vi "DopplerScale.vi"(6 "FFT Length":i32=512, 7 "Header In":T2={"header info"={"Header"="", "Head length"=0}, "A/D info"={"# rf points per line"=0, "# lines per scan"=0, "sample rate MHz"=0, "# A/D bits"=0, "# bytes per A/D"=0, "TGC Flag"=0, "A/D Type"=""}, "Tranducer Info"={"bandwidth"=0.0, "center freq"=0.0, "start freq"=0.0, "ID"=0}, "Scan Info"={"delay"=0.0, "pivot distance"=0.0, "sector scan angle"=0.0, "operator"="", "Scan Mode"="", "location"=""}, "Time/Date Info"={"date"="", "time"=""}, "RF Info"={"RF file name"="", "RF file att"="", "RF cal file name"="", "RF cal file att"=""}, "Patient Info"={"ID"="", "extended ID"="", "age"=0, "sex"="", "previously\nscanned"="", "PSA"=0.0, "LOS"=1, "Ethnicty 2"=3, "Race"=3}, "Tissue Type"={"organ"=0, "disease type"=0, "disease location"=0, "IQ_pts"=0, "RcvBuffer"=0, "RcvFrame"=0, "IQBuff"=0, "IQFrame"=0, "IQPage"=0}, "Votage scaling"={"Digitizer (dB)"=0.0, "Gain (dB)"=0.0, "Atten (dB)"=0.0}, "Comment"="", "Misc Info"={"avg num"=0, "c speed"=0, "Div By or SF zones"=0, "XMIT CHS"=0, "RCV CHS"=0, "Xmit angle"=0.0}, "Therapy Parameters"={"Theraputic Freq (MHz)"=0.0, "Time on (s)"=0.0, "Therapy amplitude (mV)"=0.0, "Lines Before"=0, "Lines After"=0}, "Scan Settings"={"Energy (uJ or V)"=0, "Damp (Ohm) or Fc"=0, "HP Filt (KHz)"=0, "LP Filt (MHz)"=0, "Gain (db)"=0, "prf (kHz)"=0.0, "Distance between\nscan lines (um)"=0, "Distance between\nscan planes (um)"=0, "Scan line gap (um)"=0.0, "Scan plane gap (um)"=0.0}, "Compression Parameters"={"F1 (MHz)"=0.0, "F2 (MHz)"=0.0, "% taper"=0.0, "duration"=0.0}, "Patient Info Xtra"={"First Name"="", "Last Name"="", "Notes"=""}, "ROI Box"=[0, 0, 0, 0]} {"Compression Parameters"."% taper" min=50 max=1000 format="%.2f"; "Compression Parameters"."F2 (MHz)" format="%.3f"; "Compression Parameters"."F1 (MHz)" format="%.3f"; "Scan Settings"."prf (kHz)" format="%.2f"; "Therapy Parameters"."Therapy amplitude (mV)" min=50 max=1000 format="%.2f"; "Therapy Parameters"."Time on (s)" format="%.3f"; "Therapy Parameters"."Theraputic Freq (MHz)" format="%.3f"; "Patient Info"."Race" items=["Am Ind or Alaska", "Asian", "Hawaiian, Pac Isl", "Black or Afr Amer", "White", "more than one race", "unknown"]; "Patient Info"."Ethnicty 2" items=["Hispanic", "Non-Hispanic", "unknown"]; "Patient Info"."LOS" items=["1", "2", "3", "4", "5"]; "Patient Info"."PSA" format="%.1f"; "Scan Info"."delay" format="%.2f"; "Scan Info"."pivot distance" format="%.2f"; "Scan Info"."sector scan angle" format="%.2f"; "Tranducer Info"."bandwidth" format="%.2f"; "Tranducer Info"."center freq" format="%.2f"; "Tranducer Info"."start freq" format="%.2f"}, 8 "Index(F)/Fd":bool, 9 "PRF1/2":bool=TRUE, 10 "Angle":dbl, 11 "Velocity index in":dbl[][](array[numeric])=array400x128[51200 elements]) -> (0 "output cluster":T1, 1 "slow-time sampling":dbl, 2 "max doppler velocity cm/s":dbl, 3 "Velocity Out":dbl[][](array[numeric]))   [LabVIEW 2022 SP3]
uses:
  Header.ctl
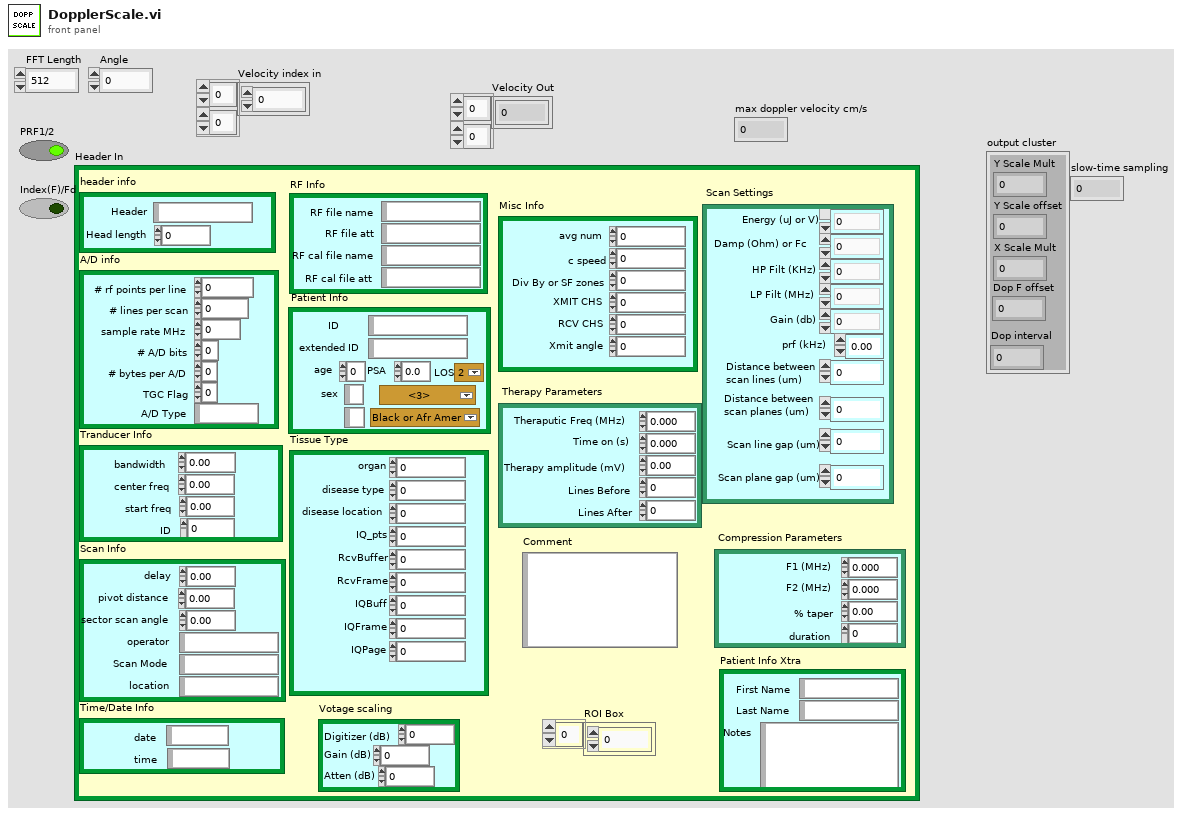
[diagram p1: front panel]
types:
  T1 = cluster{"Y Scale Mult":dbl, "Y Scale offset":dbl, "X Scale Mult":dbl, "Dop F offset":dbl, "Dop interval":dbl}
  T2 = typedef "Header.ctl" = cluster{"header info":cluster{"Header":string, "Head length":i16}, "A/D info":cluster{"# rf points per line":u16, "# lines per scan":u16, "sample rate MHz":u16, "# A/D bits":i16, "# bytes per A/D":u16, "TGC Flag":u16, "A/D Type":string}, "Tranducer Info":cluster{"bandwidth":sgl, "center freq":sgl, "start freq":sgl, "ID":i32}, "Scan Info":cluster{"delay":sgl, "pivot distance":sgl, "sector scan angle":sgl, "operator":string, "Scan Mode":string, "location":string}, "Time/Date Info":cluster{"date":string, "time":string}, "RF Info":cluster{"RF file name":string, "RF file att":string, "RF cal file name":string, "RF cal file att":string}, "Patient Info":cluster{"ID":string, "extended ID":string, "age":u16, "sex":string, "previously\nscanned":string, "PSA":sgl, "LOS":u8, "Ethnicty 2":u8, "Race":u8}, "Tissue Type":cluster{"organ":i16, "disease type":i16, "disease location":i16, "IQ_pts":u16, "RcvBuffer":u8, "RcvFrame":u16, "IQBuff":u8, "IQFrame":u16, "IQPage":u8}, "Votage scaling":cluster{"Digitizer (dB)":sgl, "Gain (dB)":sgl, "Atten (dB)":sgl}, "Comment":string, "Misc Info":cluster{"avg num":u16, "c speed":i16, "Div By or SF zones":i16, "XMIT CHS":u8, "RCV CHS":u8, "Xmit angle":sgl}, "Therapy Parameters":cluster{"Theraputic Freq (MHz)":sgl, "Time on (s)":sgl, "Therapy amplitude (mV)":sgl, "Lines Before":u16, "Lines After":u16}, "Scan Settings":cluster{"Energy (uJ or V)":u8, "Damp (Ohm) or Fc":u8, "HP Filt (KHz)":u8, "LP Filt (MHz)":u8, "Gain (db)":u8, "prf (kHz)":sgl, "Distance between\nscan lines (um)":u16, "Distance between\nscan planes (um)":u16, "Scan line gap (um)":sgl, "Scan plane gap (um)":sgl}, "Compression Parameters":cluster{"F1 (MHz)":sgl, "F2 (MHz)":sgl, "% taper":sgl, "duration":sgl}, "Patient Info Xtra":cluster{"First Name":string, "Last Name":string, "Notes":string}, "ROI Box":u16[]}
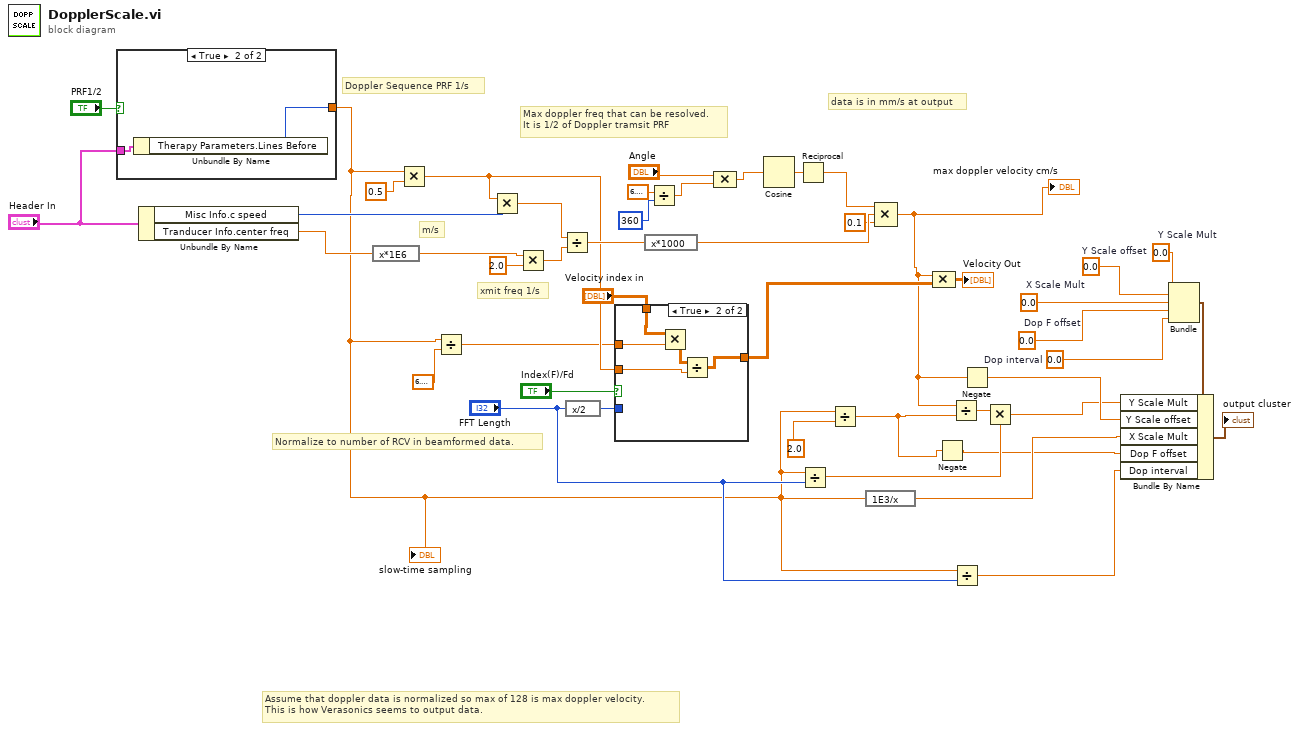
[diagram p0: block diagram]
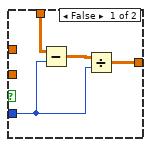
[diagram p2: hidden frame]
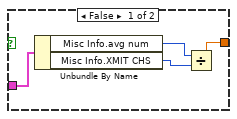
[diagram p3: hidden frame]
diagram:
  w11 = 0.0  # Dop interval
  w12 = 0.0  # Dop F offset
  w30 = 0.0  # X Scale Mult
  w31 = 0.0  # Y Scale offset
  w32 = 0.0  # Y Scale Mult
  # "Normalize to number of RCV in beamformed data."
  # "Max doppler freq that can be resolved.\nIt is 1/2 of Doppler tramsit PRF"
  # "data is in mm/s at output"
  # "Assume that doppler data is normalized so max of 128 is max doppler velocity.\nThis is how Verasonics seems to output data."
  # "m/s"
  # "xmit freq 1/s"
  # "Doppler Sequence PRF 1/s"
  n1 = case shown="True" "PRF1/2" {
    tunnel: "Header In" -> [w50 w52]
    tunnel: [w47 w51] -> w2
    frame False {
      n2 = Unbundle By Name(w50) -> ("Misc Info.avg num"=w48:u16, "Misc Info.XMIT CHS"=w49:u8)
      n3 = Divide(x=w48, y=w49) -> (x/y=w47:dbl)
    }
    frame True {
      n4 = Unbundle By Name(w52) -> ("Therapy Parameters.Lines Before"=w51:u16)
    }
  }
  "slow-time sampling" <- w2
  n5 = Unbundle By Name("Header In") -> ("Misc Info.c speed"=w45:i16, "Tranducer Info.center freq"=w42:sgl)
  n6 = expression code="x*1E6"(w42) -> (w41:sgl)
  n7 = Multiply(x=w2, y=0.5) -> (x*y=w5:dbl)
  n8 = Divide(x=w2, y=6.283185307179586) -> (x/y=w3:dbl)
  n9 = Multiply(x=w5, y=w45) -> (x*y=w37:dbl)
  n10 = Multiply(x=w41, y=2.0) -> (x*y=w44:dbl)
  n11 = Divide(x=w37, y=w44) -> (x/y=w40:dbl)
  n12 = expression code="x/2"("FFT Length") -> (w23:i32)
  n13 = case shown="True" "Index(F)/Fd" {
    tunnel: [w55 w61] -> w24
    tunnel: w23 -> [w54 _]
    tunnel: "Velocity index in" -> [w53 w58]
    tunnel: w5 -> [_ w60]
    tunnel: w3 -> [_ w59]
    frame False {
      n14 = Subtract(x=w53, y=w54) -> (x-y=w56:dbl[][])
      n15 = Divide(x=w56, y=w54) -> (x/y=w55:dbl[][])
    }
    frame True {
      n16 = Multiply(x=w58, y=w59) -> (x*y=w57:dbl[][])
      n17 = Divide(x=w57, y=w60) -> (x/y=w61:dbl[][])
    }
  }
  n18 = expression code="x*1000"(w40) -> (w21:dbl)
  n19 = Divide(x=6.283185307179586, y=360) -> (x/y=w17:dbl)
  n20 = Compound Arithmetic op=MULTIPLY("Angle", w17) -> (w15:dbl)
  n21 = Cosine(x=w15) -> (cos(x)=w20:dbl)
  n22 = Reciprocal(x=w20) -> (1/x=w14:dbl)
  n23 = Divide(x=w2, y="FFT Length") -> (x/y=w33:dbl)
  n24 = Divide(x=w2, y=2.0) -> (x/y=w8:dbl)
  n25 = expression code="1E3/x"(w2) -> (w26:dbl)
  n26 = Compound Arithmetic op=MULTIPLY(w14, w21, 0.1 ("value")) -> (w13:dbl)
  "max doppler velocity cm/s" <- w13
  n27 = Compound Arithmetic op=MULTIPLY(w13, w24) -> (→"Velocity Out":dbl[][])
  n28 = Negate(x=w8) -> (-x=w7:dbl)
  n29 = Divide(x=w13, y=w8) -> (x/y=w34:dbl)
  n30 = Divide(x=w2, y="FFT Length") -> (x/y=w9:dbl)
  n31 = Negate(x=w13) -> (-x=w28:dbl)
  n32 = Multiply(x=w34, y=w33) -> (x*y=w27:dbl)
  n33 = Bundle("Y Scale Mult"=w32, "Y Scale offset"=w31, "X Scale Mult"=w30, "Dop F offset"=w12, "Dop interval"=w11) -> (w29:T1)  [unwired: 1 in]
  n34 = Bundle By Name(cluster=w29, "Y Scale Mult"=w27, "Y Scale offset"=w28, "X Scale Mult"=w26, "Dop F offset"=w7, "Dop interval"=w9) -> (→"output cluster":T1)
